vi "Image_Crop_Fixed_Area.vi"(8 "Particle Measurements in":dbl[][](array[numeric]), 9 "Image  in":T1, 10 "SystemVersion":u16, 11 "Object size threshold":i32=500) -> (0 "Object accept":bool, 1 "Object":bool, 3 "Crop coordinates array":i32[](array[numeric]), 4 "error out":errorcluster={"status"=TRUE, "code"=-1074396120, "source"="IMAQ Get Image Size\n  "})   [LabVIEW 2024]
uses:
  <vilib>/vision/Image Controls.llb/IMAQ Image.ctl
panel:
  out "detectImg":bool
  out "Object size threshold 2":i32
  out "imgBorder":i32[](array[numeric])
  out "maxVal":i32
  out "Centroid":i32
  out "BR":i32
  out "TL":i32
  out "Image size/2":i32
  out "Max x":i32
  out "Max y":i32
  in  "Image Border":i32=20
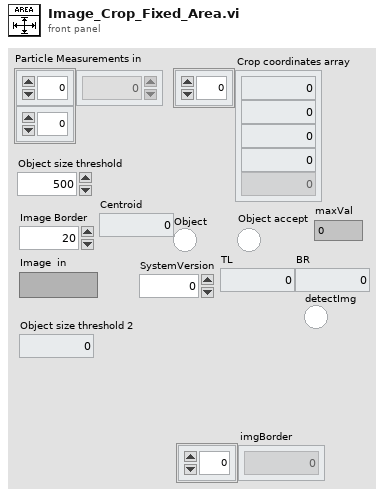
[diagram p1: front panel]
types:
  T1 = typedef "IMAQ Image.ctl" = refnum<image>
  T2 = typedef "Particle Parameters" = i32
  T3 = cluster{"Global Rectangle":i32[], "Contours":cluster{"ID":enum32{"External", "Internal"}, "Type":u32, "Coordinates":i32[]}[]}
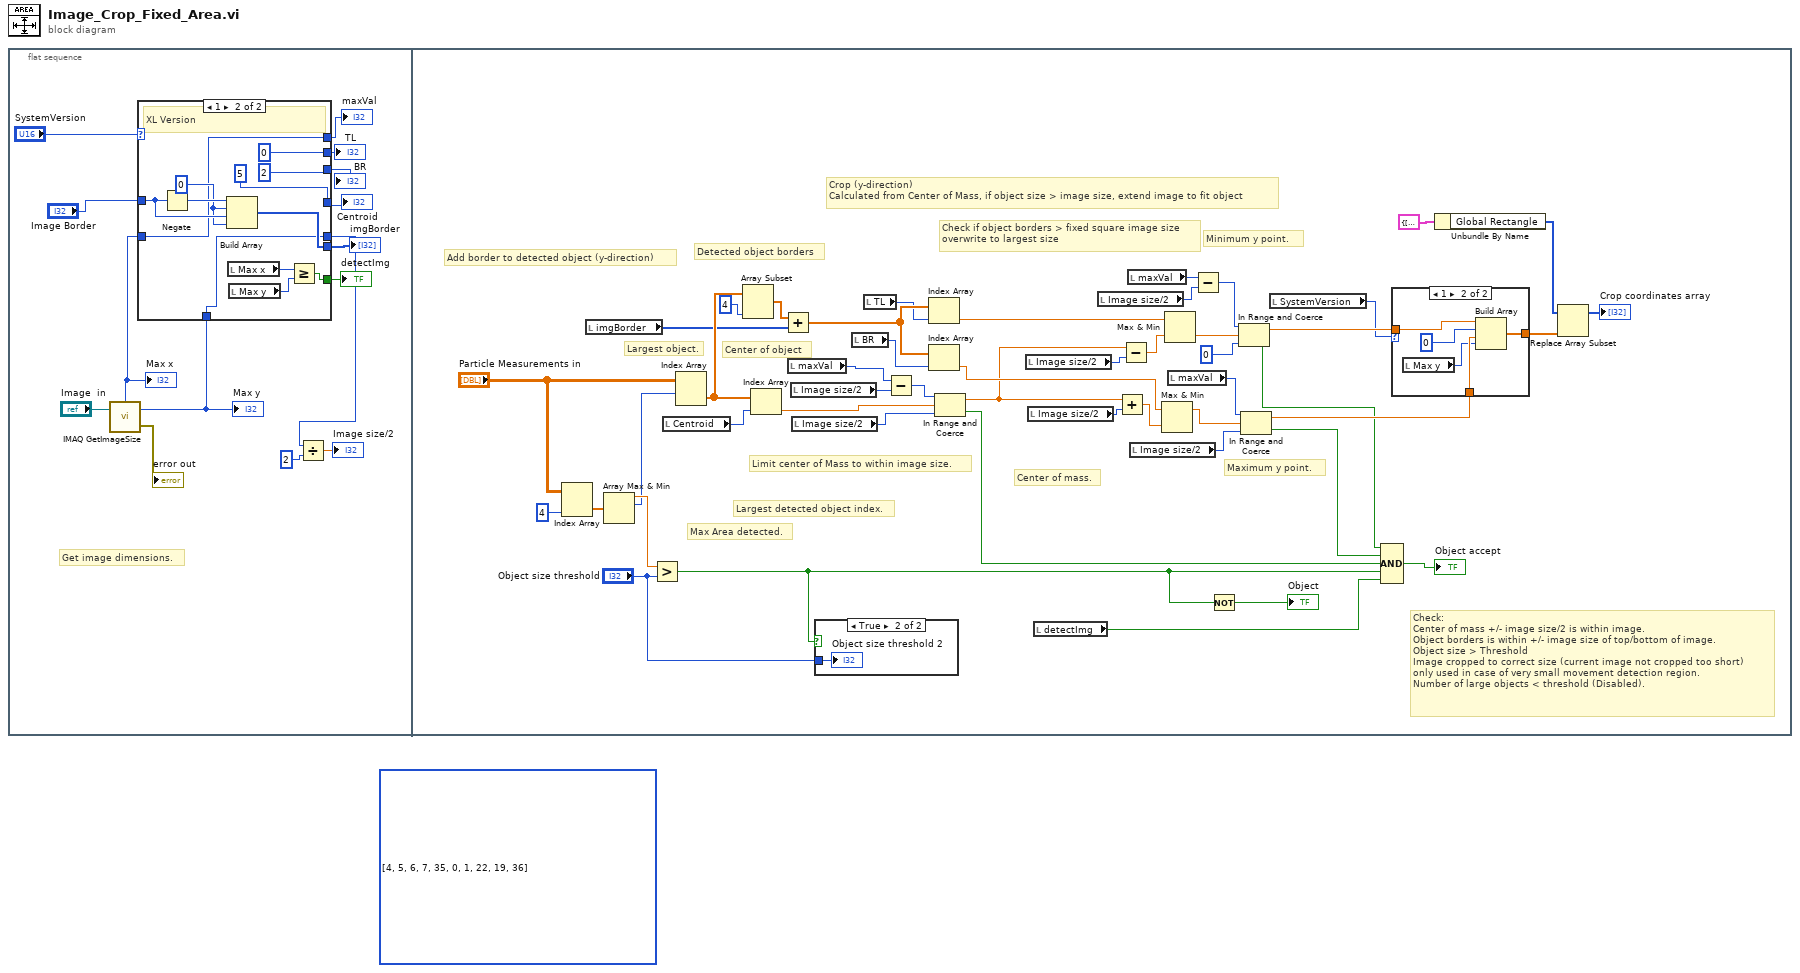
[diagram p0: block diagram]
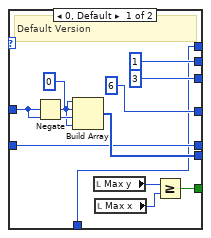
[diagram p2: hidden frame]
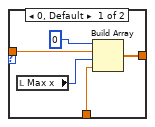
[diagram p4: hidden frame]
diagram:
  (unwired) T2[] [4, 5, 6, 7, 35, 0, 1, 22, 19, 36] items=["Center of Mass X", "Center of Mass Y", "First Pixel X", "First Pixel Y", "Bounding Rect Left", "Bounding Rect Top", "Bounding Rect Right", "Bounding Rect Bottom", "Max Feret Diameter Start X", "Max Feret Diameter Start Y", "Max Feret Diameter End X", "Max Feret Diameter End Y", "Max Horiz. Segment Length Left", "Max Horiz. Segment Length Right", "Max Horiz. Segment Length Row", "-", "Bounding Rect Width", "Bounding Rect Height", "Bounding Rect Diagonal", "Perimeter", "Convex Hull Perimeter", "Holes' Perimeter", "Max Feret Diameter", "Equivalent Ellipse Major Axis", "Equivalent Ellipse Minor Axis", "Equivalent Ellipse Minor Axis (Feret)", "Equivalent Rect Long Side", "Equivalent Rect Short Side", "Equivalent Rect Diagonal", "Equivalent Rect Short Side (Feret)", "Average Horiz. Segment Length", "Average Vert. Segment Length", "Hydraulic Radius", "Waddel Disk Diameter", "-", "Area", "Holes' Area", "Particle & Holes' Area", "Convex Hull Area", "Image Area", "-", "Number of Holes", "Number of Horiz. Segments", "Number of Vert. Segments", "-", "Orientation", "Max Feret Diameter Orientation", "-", "% Area/Image Area", "% Area/(Particle & Holes' Area)", "Ratio of Equivalent Ellipse Axes", "Ratio of Equivalent Rect Sides", "-", "Elongation Factor", "Compactness Factor", "Heywood Circularity Factor", "Type Factor", "-", "Sum X", "Sum Y", "Sum XX", "Sum XY", "Sum YY", "Sum XXX", "Sum XXY", "Sum XYY", "Sum YYY", "-", "Moment of Inertia XX", "Moment of Inertia XY", "Moment of Inertia YY", "Moment of Inertia XXX", "Moment of Inertia XXY", "Moment of Inertia XYY", "Moment of Inertia YYY", "Norm. Moment of Inertia XX", "Norm. Moment of Inertia XY", "Norm. Moment of Inertia YY", "Norm. Moment of Inertia XXX", "Norm. Moment of Inertia XXY", "Norm. Moment of Inertia XYY", "Norm. Moment of Inertia YYY", "Hu Moment 1", "Hu Moment 2", "Hu Moment 3", "Hu Moment 4", "Hu Moment 5", "Hu Moment 6", "Hu Moment 7"] ("Pixel Measurements")
  n1 = flat-sequence {
    frame #0 {
      # "Get image dimensions."
      n2 = call "IMAQ GetImageSize"("Image"="Image  in") -> ("Y Resolution"=w7:i32, "X Resolution"=w6:i32, "error out"=→"error out":errorcluster)  [unwired: 3 in]
      "Max y" <- w7
      "Max x" <- w6
      n3 = case shown="1" "SystemVersion" {
        tunnel: [1 ("index") 0 ("index")] -> w10
        tunnel: [3 ("index") 2 ("index")] -> w9
        tunnel: [6 ("index") 5 ("index")] -> w8
        tunnel: [w17 w28] -> w5
        tunnel: w7 -> [w16 w28]
        tunnel: w6 -> [w17 w29]
        tunnel: [w16 w29] -> w4
        tunnel: "Image Border" -> [w22 w35]
        tunnel: [w24 w33] -> w2
        tunnel: [w18 w30] -> w1
        frame 0, Default {
          w21 = 0 ("element")
          # "Default Version"
          n4 = Negate(x=w22) -> (-x=w23:i32)
          n5 = Build Array(w23, w21, w22, w21) -> (w24:i32[])
          n6 = local read "Max y"() -> (w20:i32)
          n7 = local read "Max x"() -> (w19:i32)
          n8 = Greater Or Equal?(x=w20, y=w19) -> (x >= y?=w18:bool)
        }
        frame 1 {
          w34 = 0 ("element")
          # "XL Version"
          n9 = Negate(x=w35) -> (-x=w36:i32)
          n10 = Build Array(w36, w34, w35, w34) -> (w33:i32[])
          n11 = local read "Max x"() -> (w32:i32)
          n12 = local read "Max y"() -> (w31:i32)
          n13 = Greater Or Equal?(x=w32, y=w31) -> (x >= y?=w30:bool)
        }
      }
      "TL" <- w10
      "BR" <- w9
      "Centroid" <- w8
      "maxVal" <- w4
      "imgBorder" <- w2
      "detectImg" <- w1
      n14 = Divide(x=w5, y=2) -> (x/y=→"Image size/2":dbl)
    }
    frame #1 {
      # "Largest object."
      # "Check:\nCenter of mass +/- image size/2 is within image.\nObject borders is within +/- image size of top/bottom of image.\nObject size > Threshold\nImage cropped to correct size (current image not cropped too short)\nonly used in case of very small movement detection region.\nNumber of large objects < threshold (Disabled)."
      # "Max Area detected."
      # "Maximum y point."
      # "Minimum y point."
      # "Center of mass."
      # "Limit center of Mass to within image size."
      # "Add border to detected object (y-direction)"
      # "Largest detected object index."
      # "Check if object borders > fixed square image size\noverwrite to largest size"
      # "Detected object borders"
      # "Center of object"
      # "Crop (y-direction)\nCalculated from Center of Mass, if object size > image size, extend image to fit object"
      n15 = Index Array(array="Particle Measurements in", index (col)=4 ("index (row)")) -> (element=w51:dbl[])  [unwired: 1 in]
      n16 = local read "imgBorder"() -> (w43:i32[])
      n17 = Array Max & Min(array=w51) -> (max value=w83:dbl, max index (indices)=w81:i32)  [unwired: 2 out]
      n18 = Greater?(x=w83, y="Object size threshold") -> (0:w42:bool)
      n19 = local read "Centroid"() -> (w49:i32)
      n20 = Index Array(array="Particle Measurements in", index (row)=w81) -> (element=w54:dbl[])  [unwired: 1 in]
      n21 = Array Subset(array=w54, length=4) -> (w79:dbl[])  [unwired: 1 in]
      n22 = Index Array(array=w54, index=w49) -> (element=w70:dbl)
      n23 = Add(x=w79, y=w43) -> (x+y=w53:dbl[])
      n24 = local read "maxVal"() -> (w46:i32)
      n25 = local read "Image size/2"() -> (w75:i32)
      n26 = local read "Image size/2"() -> (w68:i32)
      n27 = case shown="True" w42 {
        tunnel: "Object size threshold" -> [_ w88]
        frame False {
        }
        frame True {
          "Object size threshold 2" <- w88
        }
      }
      n28 = local read "BR"() -> (w47:i32)
      n29 = local read "TL"() -> (w48:i32)
      n30 = Subtract(x=w46, y=w75) -> (x-y=w69:i32)
      n31 = Index Array(array=w53, index=w48) -> (element=w78:dbl)
      n32 = Index Array(array=w53, index=w47) -> (element=w77:dbl)
      n33 = In Range and Coerce(upper limit=w69, x=w70, lower limit=w68) -> (coerced(x)=w66:dbl, In Range?=w67:bool)
      n34 = local read "Image size/2"() -> (w72:i32)
      n35 = local read "Image size/2"() -> (w71:i32)
      n36 = local read "detectImg"() -> (w40:bool)
      n37 = local read "Image size/2"() -> (w62:i32)
      n38 = Add(x=w66, y=w71) -> (x+y=w74:dbl)
      n39 = Subtract(x=w66, y=w72) -> (x-y=w73:dbl)
      n40 = local read "maxVal"() -> (w44:i32)
      n41 = local read "Image size/2"() -> (w60:i32)
      n42 = Max & Min(x=w77, y=w74) -> (max(x,y)=w55:dbl)  [unwired: 1 out]
      n43 = Max & Min(x=w78, y=w73) -> (min(x,y)=w65:dbl)  [unwired: 1 out]
      n44 = local read "maxVal"() -> (w45:i32)
      n45 = Subtract(x=w44, y=w62) -> (x-y=w61:i32)
      n46 = Not(x=w42) -> (.not. x?=→"Object":bool)
      n47 = In Range and Coerce(upper limit=w61, x=w65, lower limit=0 ("x")) -> (coerced(x)=w63:dbl, In Range?=w57:bool)
      n48 = In Range and Coerce(upper limit=w45, x=w55, lower limit=w60) -> (coerced(x)=w59:dbl, In Range?=w58:bool)
      n49 = local read "SystemVersion"() -> (w50:u16)
      n50 = Compound Arithmetic op=AND(w57, w58, w67, w42, w40) -> (→"Object accept":bool)
      n51 = case shown="1" w50 {
        tunnel: [w93 w98] -> w76
        tunnel: w63 -> [w90 w97]
        tunnel: w59 -> [w89 w95]
        frame 0, Default {
          n52 = local read "Max x"() -> (w91:i32)
          n53 = Build Array(0 ("x"), w90, w91, w89) -> (w93:dbl[])
        }
        frame 1 {
          n54 = local read "Max y"() -> (w94:i32)
          n55 = Build Array(w97, 0 ("x"), w95, w94) -> (w98:dbl[])
        }
      }
      n56 = Unbundle By Name(T3 {"Global Rectangle"=[106, 29, 356, 265], "Contours"=[{"ID"=enum."External", "Type"=3, "Coordinates"=[106, 29, 356, 265]}]} ("Crop to object")) -> ("Global Rectangle"=w87:i32[])
      n57 = Replace Array Subset(array=w87, new element=w76) -> (→"Crop coordinates array":i32[])  [unwired: 1 in]
    }
  }
